vi "gu_reverse_string.vi"(8 "error in":errorcluster, 11 "Encoded String in":T1) -> (0 "error out":errorcluster, 3 "Encoded String out":string)   [LabVIEW 2020, in "G-Unicode.lvlib"]
uses:
  G-Unicode.lvlib
  lib/g_unicode_32.dll
  Types/Encoded UTF-8 String.ctl
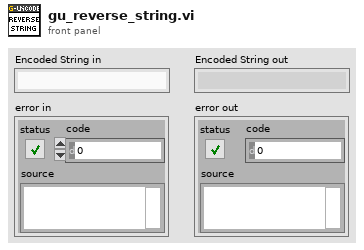
[diagram p1: front panel]
types:
  T1 = typedef "G-Unicode.lvlib/Encoded UTF-8 String.ctl" = string
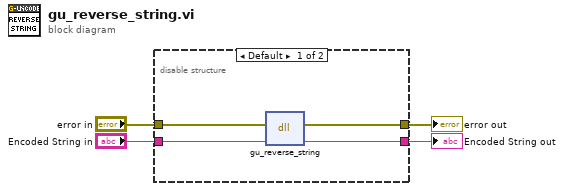
[diagram p0: block diagram]
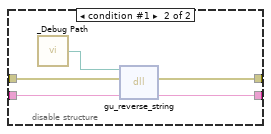
[diagram p2: hidden frame]
diagram:
  n1 = disable-structure shown="Default" {
    disable-tunnel: "Encoded String in" -> [w8 w13]
    disable-tunnel: "error in" -> [w7 w12]
    disable-tunnel: [w6 w11] -> w2
    disable-tunnel: [w5 w10] -> w1
    frame condition #0 (active) {
      n2 = dll-call lib="C:/github/dataflowg/g-unicode/src/LabVIEW/G-Unicode/lib/g_unicode_*.*" fn="gu_reverse_string"(error in=w7, "str"=w8) -> (error out=w6:errorcluster, "str"=w5:string)  [unwired: 3 in, 1 out]
    }
    frame condition #1 {
      n3 = call "_Debug Path.vi"() -> ("Debug Path"=w9:path)
      n4 = dll-call lib="?" fn="gu_reverse_string"(path in=w9, error in=w12, "str"=w13) -> (error out=w11:errorcluster, "str"=w10:string)  [unwired: 2 in, 1 out]
    }
  }
  "error out" <- w2
  "Encoded String out" <- w1
